vi "OAT Edge Detection (1 Tach).vi"(5 "reset? (True)":bool=TRUE, 6 "sampling frequency [Hz]":dbl=11025.0, 7 "missing pulses? (no:F)":bool, 8 "slope (Rising)":u16(ring) items=["Rising", "Falling"], 9 "pulse width (2)":i32=2, 10 "threshold (0.0)":dbl format="%.2f", 11 "x[n]":dbl[](array[numeric]) format="%.2f") -> (1 "number of pulses":i32, 3 "pulse positions [s]":dbl[](array[numeric]) format="%.2f")   [LabVIEW 2017, in "SoundVib_TachProcess.lvlib"]
doc: "Detects the edges in the tachometer pulses contained in <B>x[n]</B> that cross <B>threshold</B>. Perform edge detection to determine the tachometer pulse position. The VI recognizes the points where the signal crosses <B>threshold</B> and <B>x[n]</B> as edges. The VI returns the locations of the detected edges in <B>pulse positions [s]</B>."
uses:
  <vilib>/addons/Sound and Vibration/Order Analysis/Tach Process/SoundVib_TachProcess.lvlib
  <vilib>/Analysis/8numeric.llb/Threshold Detector.vi
panel:
  # "Edge Detection (1 Tach)"
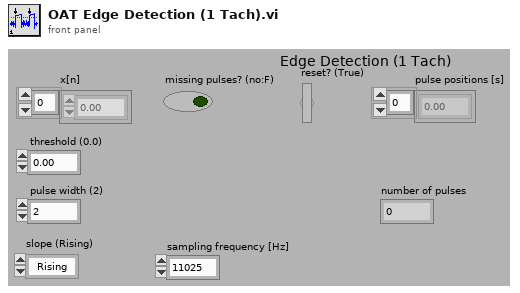
[diagram p1: front panel]
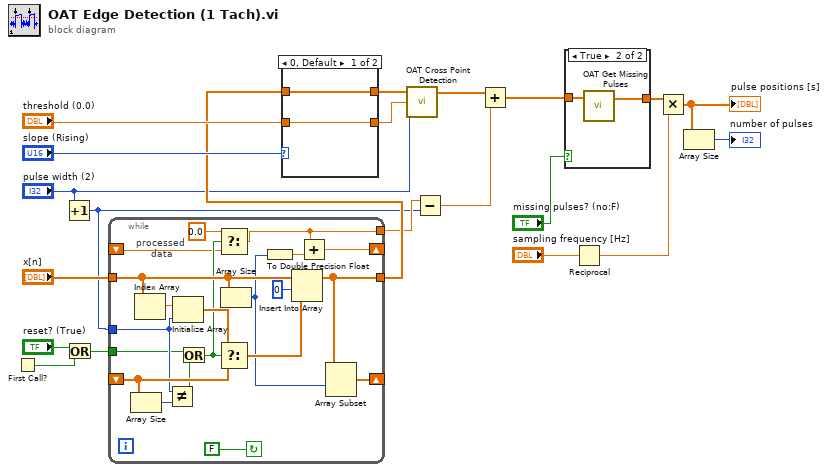
[diagram p0: block diagram]
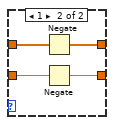
[diagram p3: hidden frame]
diagram:
  n1 = First Call?() -> (First Call?: T/F=w2:bool)
  n2 = Increment(x="pulse width (2)") -> (x+1=w1:i32)
  n3 = Or(x="reset? (True)", y=w2) -> (x .or. y?=w10:bool)
  n4 = while {
    shift-right: [w34] -> _
    shift-left: _ -> [w39]
    tunnel: "x[n]" -> [w33]
    tunnel: w1 -> [w37]
    tunnel: [w30] -> w11
    tunnel: w10 -> [w35]
    shift-right: [w29] -> _
    shift-left: _ -> [w26]
    tunnel: [w24] -> w7
    stop <- FALSE continue-if-true
    # "processed\n     data"
    n5 = Array Size(array=w39) -> (size(s)=w38:i32)
    n6 = Index Array(array=w33) -> (element=w40:dbl)  [unwired: 1 in]
    n7 = Not Equal?(x=w37, y=w38) -> (x != y?=w36:bool)
    n8 = Initialize Array(w40, w37) -> (w28:dbl[])
    n9 = Or(x=w35, y=w36) -> (x .or. y?=w27:bool)
    n10 = Select(t=0.0, s=w27, f=w26) -> (s? t:f=w24:dbl)
    n11 = Select(t=w28, s=w27, f=w39) -> (s? t:f=w32:dbl[])
    n12 = Array Size(array=w33) -> (size(s)=w23:i32)
    n13 = To Double Precision Float(number=w23) -> (double precision float=w22:dbl)
    n14 = Insert Into Array(array=w33, index=0 ("Index"), new element=w32) -> (w30:dbl[])
    n15 = Add(x=w24, y=w22) -> (x+y=w29:dbl)
    n16 = Array Subset(array=w30, index=w23) -> (w34:dbl[])  [unwired: 1 in]
  }
  n17 = case shown="0, Default" "slope (Rising)" {
    tunnel: "threshold (0.0)" -> [w42 w45]
    tunnel: w11 -> [w43 w47]
    tunnel: [w43 w46] -> w18
    tunnel: [w42 w44] -> w20
    frame 0, Default {
    }
    frame 1 {
      n18 = Negate(x=w47) -> (-x=w46:dbl[])
      n19 = Negate(x=w45) -> (-x=w44:dbl)
    }
  }
  n20 = call <vilib>:"OAT Cross Point Detection.vi"("pulse width (2)"="pulse width (2)", "threshold (0)"=w20, "data in"=w18) -> ("edge position"=w8:dbl[])  [unwired: 1 in]
  n21 = Subtract(x=w7, y=w1) -> (x-y=w5:dbl)
  n22 = Add(x=w8, y=w5) -> (x+y=w9:dbl[])
  n23 = case shown="True" "missing pulses? (no:F)" {
    tunnel: w9 -> [w48 w50]
    tunnel: [w48 w49] -> w16
    frame False {
    }
    frame True {
      n24 = call <vilib>:"OAT Get Missing Pulses.vi"("pulse positions"=w50) -> ("modified pulse positions"=w49:dbl[])  [unwired: 1 in, 1 out]
    }
  }
  n25 = Reciprocal(x="sampling frequency [Hz]") -> (1/x=w4:dbl)
  n26 = Multiply(x=w16, y=w4) -> (x*y=w14:dbl[])
  "pulse positions [s]" <- w14
  n27 = Array Size(array=w14) -> (size(s)=→"number of pulses":i32)
